vi "New (Array).vi"(8 "error in (no error)":errorcluster, 9 "aggregation method (all)":T2=enum."All", 10 "match behavior (keep)":T1, 11 "data item names":string[](array[string])) -> (0 "error out":errorcluster, 3 "data item out":refnum<class "Data Item.lvclass">)   [LabVIEW 2018, in "GLog.lvlib" / "Data Item.lvclass"]
uses:
  Data Item.lvclass
  C:/Users/Colin/Documents/software_projects/glog/src/api/extension/filter_interface/Filter.lvclass
  extension/filter_interface/Aggregation Method.ctl
  extension/filter_interface/Match Behavior.ctl
  Data Item.lvclass/Data Item.ctl
  extension/filter_interface/Filter.lvclass/Filter.ctl
  extension/filter_interface/Filter.lvclass
  GLog.lvlib
panel:
  # "Connector Pane"
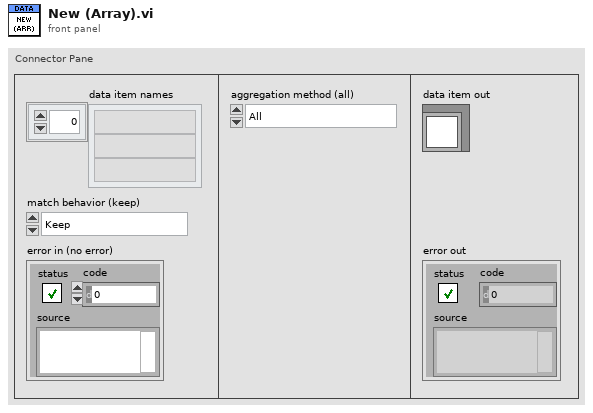
[diagram p1: front panel]
types:
  T1 = typedef "GLog.lvlib/Match Behavior.ctl" = enum16{"Keep", "Discard"}
  T2 = typedef "GLog.lvlib/Aggregation Method.ctl" = enum16{"Any", "Only", "All", "None"}
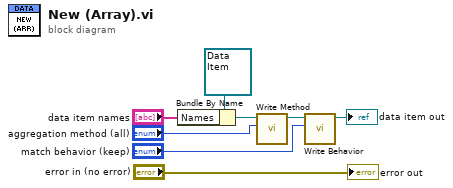
[diagram p0: block diagram]
diagram:
  n1 = Bundle By Name(cluster=refnum<class "Data Item.lvclass"> refnum ("Logging.lvlib:Data Item.lvclass"), "Names"="data item names") -> (w5:refnum<class "Data Item.lvclass">)
  n2 = call "Write Method.vi"("Method"="aggregation method (all)", "Filter in"=w5) -> ("Filter out"=w3:refnum<class "Data Item.lvclass">)  [unwired: 9 in]
  n3 = call "Write Behavior.vi"("match behavior"="match behavior (keep)", "Filter in"=w3) -> ("Filter out"=→"data item out":refnum<class "Data Item.lvclass">)  [unwired: 9 in]
  "error out" <- "error in (no error)"
